vi "Send Flight Mode Message.vi"(8 "Error In":errorcluster, 11 "Flight Mode":T1) -> (0 "Error Out":errorcluster)   [LabVIEW 2014]
uses:
  MAVLink/Controls/MAVLink Flight modes.ctl
  Aircraft Information/Sub VI/Selected Aircraft/SubVI/Get Selected Aircraft.vi
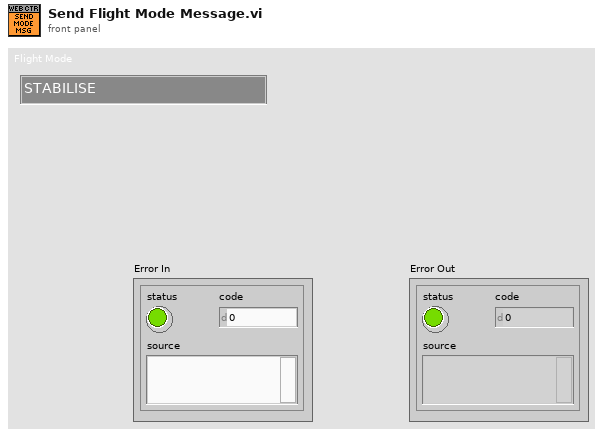
[diagram p1: front panel]
types:
  T1 = typedef "MAVLink Flight modes.ctl" = enum32{"STABILISE", "ACRO", "ALT HOLD", "AUTO", "GUIDED", "LOITER", "RTL", "CIRCLE", "UNKNOWN1", "LAND", "OF LOITER", "DRIFT", "UNKNOWN2", "SPORT", "FLIP", "AUTO TUNE", "POS HOLD", "BRAKE"}
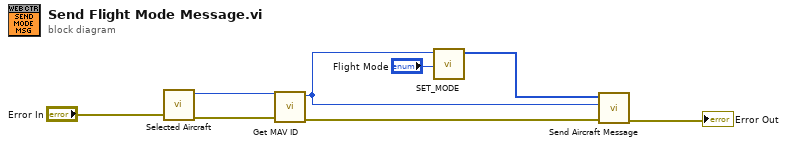
[diagram p0: block diagram]
diagram:
  n1 = call-poly "Selected Aircraft.vi"("Error In"="Error In") -> ("Error Out"=w7:errorcluster, "Selected Aircraft ID Out"=w8:u8)  [unwired: 9 in]
  n2 = call "Get MAV ID.vi"("Error In"=w7, "Aircraft Index"=w8) -> ("Error Out"=w4:errorcluster, "Aircraft ID"=w5:u8)  [unwired: 8 in]
  n3 = call "SET_MODE.vi"("Flight Mode"="Flight Mode", "target_system"=w5) -> ("MAVLink Message"=w3:u8[])  [unwired: 9 in]
  n4 = call "Send Aircraft Message.vi"("error in (no error)"=w4, "Aircraft ID"=w5, "MAVLink Message"=w3) -> ("error out"=→"Error Out":errorcluster)  [unwired: 8 in]
